vi "Ideal_counters.vi"(2 "Odour bottles":T1(array[cluster])=[[{"Mixture components"=[{"Name"="MINERAL OIL", "CID"=0, "Volatility"=0.0}], "Name"="B1 (Bl)", "VPs"="0.0E+0", "Proportion"=[{"Numeric"=100.0}], "Selected"=FALSE, "Counter"=TRUE}, {"Mixture components"=[{"Name"="Methyl benzoate", "CID"=8103, "Volatility"=0.38}, {"Name"="Menthone", "CID"=8063, "Volatility"=0.28}], "Name"="B3 (ME2)", "VPs"="3.3E-1 ± 21%", "Proportion"=[{"Numeric"=50.0}, {"Numeric"=50.0}], "Selected"=TRUE, "Counter"=FALSE}, {"Mixture components"=[{"Name"="Decanol", "CID"=460, "Volatility"=0.00851}], "Name"="B5 (C4f)", "VPs"="8.5E-3", "Proportion"=[{"Numeric"=100.0}], "Selected"=FALSE, "Counter"=FALSE}, {"Mixture components"=[{"Name"="Acetophenone", "CID"=8174, "Volatility"=0.45}, {"Name"="Fenchone", "CID"=8635, "Volatility"=0.82}], "Name"="B7 (ME1)", "VPs"="6.4E-1 ± 41%", "Proportion"=[{"Numeric"=50.0}, {"Numeric"=50.0}], "Selected"=FALSE, "Counter"=FALSE}], [{"Mixture components"=[{"Name"="MINERAL OIL", "CID"=0, "Volatility"=0.0}], "Name"="B2 (Bl)", "VPs"="0.0E+0", "Proportion"=[{"Numeric"=100.0}], "Selected"=FALSE, "Counter"=TRUE}, {"Mixture components"=[{"Name"="Octanol", "CID"=7439, "Volatility"=0.0794}], "Name"="B4 (C4cA)", "VPs"="7.9E-2", "Proportion"=[{"Numeric"=100.0}], "Selected"=FALSE, "Counter"=FALSE}, {"Mixture components"=[{"Name"="MINERAL OIL", "CID"=0, "Volatility"=0.0}], "Name"="B6 (Bl)", "VPs"="0.0E+0", "Proportion"=[{"Numeric"=100.0}], "Selected"=FALSE, "Counter"=FALSE}, {"Mixture components"=[{"Name"="Heptanoic acid ", "CID"=957, "Volatility"=0.0107}], "Name"="B8 (C3cA)", "VPs"="1.1E-2", "Proportion"=[{"Numeric"=100.0}], "Selected"=FALSE, "Counter"=FALSE}], [{"Mixture components"=[{"Name"="MINERAL OIL", "CID"=0, "Volatility"=0.0}], "Name"="B9 (Bl)", "VPs"="0.0E+0", "Proportion"=[{"Numeric"=100.0}], "Selected"=FALSE, "Counter"=TRUE}, {"Mixture components"=[{"Name"="Geranyl acetate", "CID"=6985, "Volatility"=0.03}, {"Name"="Dimethylacetophenone", "CID"=7144, "Volatility"=0.063}], "Name"="B11 (MW1)", "VPs"="4.6E-2 ± 50%", "Proportion"=[{"Numeric"=50.0}, {"Numeric"=50.0}], "Selected"=FALSE, "Counter"=FALSE}, {"Mixture components"=[{"Name"="Geraniol", "CID"=6405, "Volatility"=0.03}, {"Name"="Phenyl butanone", "CID"=7762, "Volatility"=0.1}], "Name"="B13 (MW2)", "VPs"="6.5E-2 ± 76%", "Proportion"=[{"Numeric"=50.0}, {"Numeric"=50.0}], "Selected"=FALSE, "Counter"=FALSE}, {"Mixture components"=[{"Name"="Methylheptanoic acid", "CID"=1032, "Volatility"=0.018}], "Name"="B15 (C3f)", "VPs"="1.8E-2", "Proportion"=[{"Numeric"=100.0}], "Selected"=FALSE, "Counter"=FALSE}], [{"Mixture components"=[{"Name"="MINERAL OIL", "CID"=0, "Volatility"=0.0}], "Name"="B10 (Bl)", "VPs"="0.0E+0", "Proportion"=[{"Numeric"=100.0}], "Selected"=FALSE, "Counter"=FALSE}, {"Mixture components"=[{"Name"="Valeric acid", "CID"=8025, "Volatility"=0.196}], "Name"="B12 (C3cB)", "VPs"="2.0E-1", "Proportion"=[{"Numeric"=100.0}], "Selected"=FALSE, "Counter"=FALSE}, {"Mixture components"=[{"Name"="Nonanol", "CID"=4133, "Volatility"=0.0227}], "Name"="B14 (C4cB)", "VPs"="2.3E-2", "Proportion"=[{"Numeric"=100.0}], "Selected"=FALSE, "Counter"=FALSE}, {"Mixture components"=[{"Name"="Hydroxacetophenone", "CID"=7462, "Volatility"=0.0856}], "Name"="B16 (Ol)", "VPs"="8.6E-2", "Proportion"=[{"Numeric"=100.0}], "Selected"=FALSE, "Counter"=FALSE}]], 4 "Bottle":i32=12) -> (0 "All counters":i32[](array[numeric]), 1 "Ideal counter order":i32[](array[numeric]))   [LabVIEW 2016]
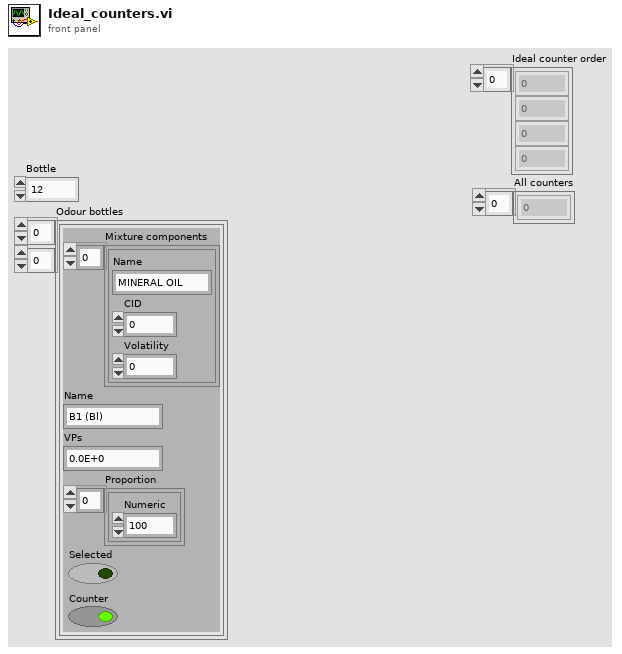
[diagram p1: front panel]
types:
  T1 = cluster{"Mixture components":cluster{"Name":string, "CID":i32, "Volatility":dbl}[], "Name":string, "VPs":string, "Proportion":cluster{"Numeric":dbl}[], "Selected":bool, "Counter":bool}[][]
  T2 = cluster{"Mixture components":cluster{"Name":string, "CID":i32, "Volatility":dbl}[], "Name":string, "VPs":string, "Proportion":cluster{"Numeric":dbl}[], "Selected":bool, "Counter":bool}[]
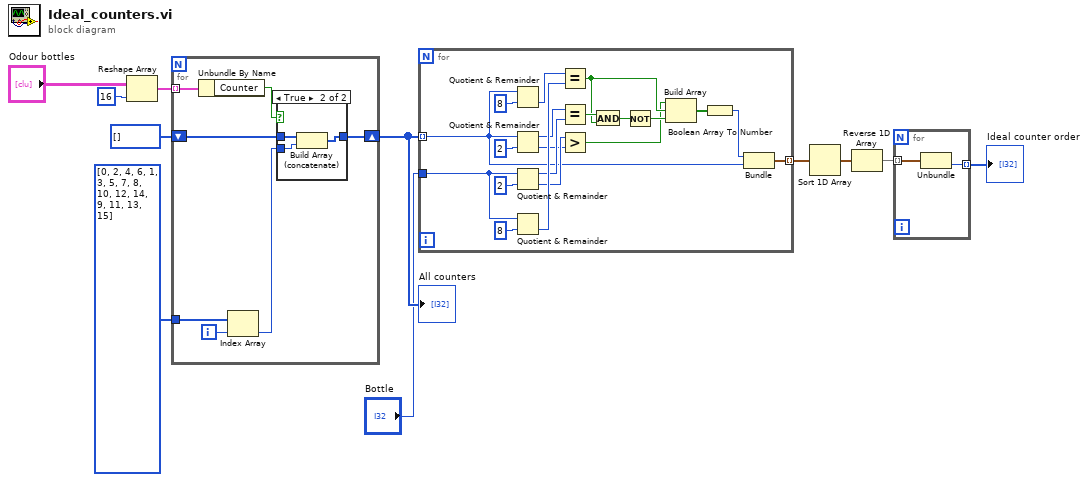
[diagram p0: block diagram]
diagram:
  n1 = Reshape Array("Odour bottles", 16 ("dimension size")) -> (w10:T2)
  n2 = for {
    tunnel: w10 -> [w18] mode=indexing
    shift-right: [w16] -> w6
    shift-left: i32[] [] -> [w17]
    tunnel: i32[] [0, 2, 4, 6, 1, 3, 5, 7, 8, 10, 12, 14, 9, 11, 13, 15] -> [w14]
    i -> [w13]
    n3 = Unbundle By Name(w18) -> ("Counter"=w15:bool)
    n4 = Index Array(array=w14, index=w13) -> (element=w12:i32)
    n5 = case shown="True" w15 {
      tunnel: w17 -> [w19 w22]
      tunnel: [w19 w21] -> w16
      tunnel: w12 -> [_ w20]
      frame False {
      }
      frame True {
        n6 = Build Array (concatenate)(w22, w20) -> (w21:i32[])
      }
    }
  }
  "All counters" <- w6
  n7 = for {
    tunnel: w6 -> [w24] mode=indexing
    tunnel: "Bottle" -> [w36]
    tunnel: [w23] -> w4 mode=indexing
    n8 = Quotient & Remainder(x=w24, y=8) -> (floor(x/y)=w40:i32)  [unwired: 1 out]
    n9 = Quotient & Remainder(x=w24, y=2) -> (x-y*floor(x/y)=w35:i32, floor(x/y)=w29:i32)
    n10 = Quotient & Remainder(x=w36, y=2) -> (x-y*floor(x/y)=w34:i32, floor(x/y)=w30:i32)
    n11 = Quotient & Remainder(x=w36, y=8) -> (floor(x/y)=w39:i32)  [unwired: 1 out]
    n12 = Equal?(x=w40, y=w39) -> (x = y?=w31:bool)
    n13 = Equal?(x=w35, y=w34) -> (x = y?=w33:bool)
    n14 = Greater?(x=w30, y=w29) -> (0:w26:bool)
    n15 = And(x=w33, y=w31) -> (x .and. y?=w32:bool)
    n16 = Not(x=w32) -> (.not. x?=w27:bool)
    n17 = Build Array(w26, w31, w27) -> (w28:bool[])
    n18 = Boolean Array To Number(Boolean array=w28) -> (number=w25:u32)
    n19 = Bundle(w25, w24) -> (w23:cluster{u32, i32})  [unwired: 1 in]
  }
  n20 = Sort 1D Array(array=w4) -> (sorted array=w3:cluster{u32, i32}[])
  n21 = Reverse 1D Array(array=w3) -> (reversed array=w2:cluster{u32, i32}[])
  n22 = for {
    tunnel: w2 -> [w44] mode=indexing
    tunnel: [w43] -> w1 mode=indexing
    n23 = Unbundle(w44) -> (w43:i32)  [unwired: 1 out]
  }
  "Ideal counter order" <- w1
